vi "GDevCon Loops.vi"() -> ()   [LabVIEW 2020, in "CTI-Scratchpad.lvlib"]
uses:
  CTI-Scratchpad.lvlib
  CTI/Error Reporting.ctl
  CTI/GPIO Number.ctl
  CTI/I2C Number.ctl
  CTI/ADC Number.ctl
  CTI-Peripheral/Character LCD/Position.ctl
  CTI/GPIO Direction.ctl
  CTI/Raw ADC.ctl
  CTI-Peripheral/Grove I2C LCD/Grove I2C LCD.lvclass
  CTI/Session/Session.lvclass
  CTI/VisaComms/VisaComms.lvclass
  CTI/CTI.lvlib
  CTI-Peripheral/Character LCD/Char LCD.lvclass
panel:
  in  "Home":bool
  in  "Clear":bool
  in  "LED":bool
  in  "PWM Enable":bool
  out "Act. Freq":sgl format="%.4f"
  out "Act. Duty":sgl format="%_6f"
  in  "Frequency":sgl(slide) scale=10.0..500000.0
  in  "Duty":sgl(slide) scale=0.0..1.0
  out "Mic":dbl(knob) scale=0.0..4095.0
  out "PIR":bool
  out "Button":bool
  in  "Position":T1
  in  "Goto":bool
  out "Potentiometer":dbl(knob) scale=0.0..1.0
  in  "Write LCD":bool
  in  "LCD Text":string
  in  "Stop":bool
  in  "I2C Baud":u32=400000 format="%.0p"
  in  "Mic AI":T2=1
  in  "Pot AI":T2
  in  "SDA GPIO":T3=6
  in  "SCL GPIO":T3=7
  in  "I2C #":T4=1
  in  "PIR GPIO":T3=28
  in  "Buzzer GPIO":T3=18
  in  "LED GPIO":T3=20
  in  "Button GPIO":T3=16
  in  "Error Checking":T5
  in  "VISA resource name":refnum<visa-resource-name>="COM5"
  # "Buzzer"
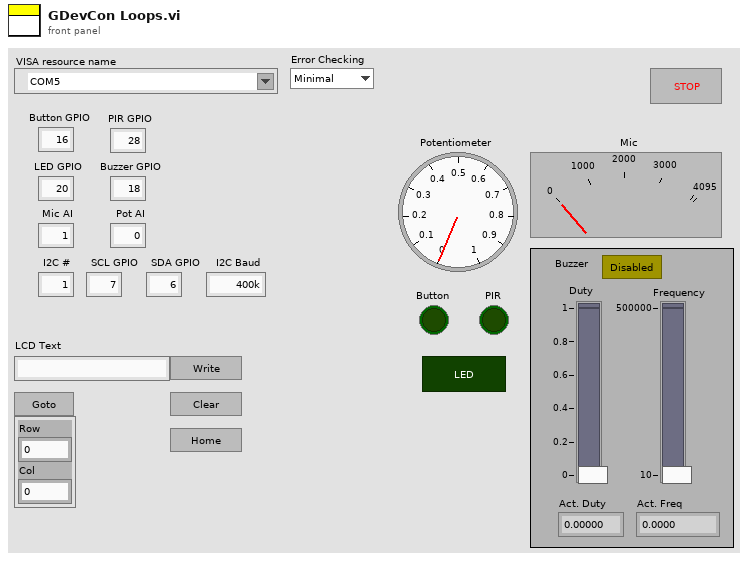
[diagram p1: front panel]
types:
  T1 = typedef "CTI-Peripheral.lvlib/Char LCD.lvclass/Position.ctl" = cluster{"Row":u8, "Col":u8}
  T2 = typedef "CTI.lvlib/ADC Number.ctl" = i8
  T3 = typedef "CTI.lvlib/GPIO Number.ctl" = i8
  T4 = typedef "CTI.lvlib/I2C Number.ctl" = i8
  T5 = typedef "CTI.lvlib/Error Reporting.ctl" = enum16{"Minimal", "Moderate", "Full"}
  T6 = typedef "CTI.lvlib/GPIO Direction.ctl" = enum16{"In", "Out"}
  T7 = typedef "CTI.lvlib/Raw ADC.ctl" = u16
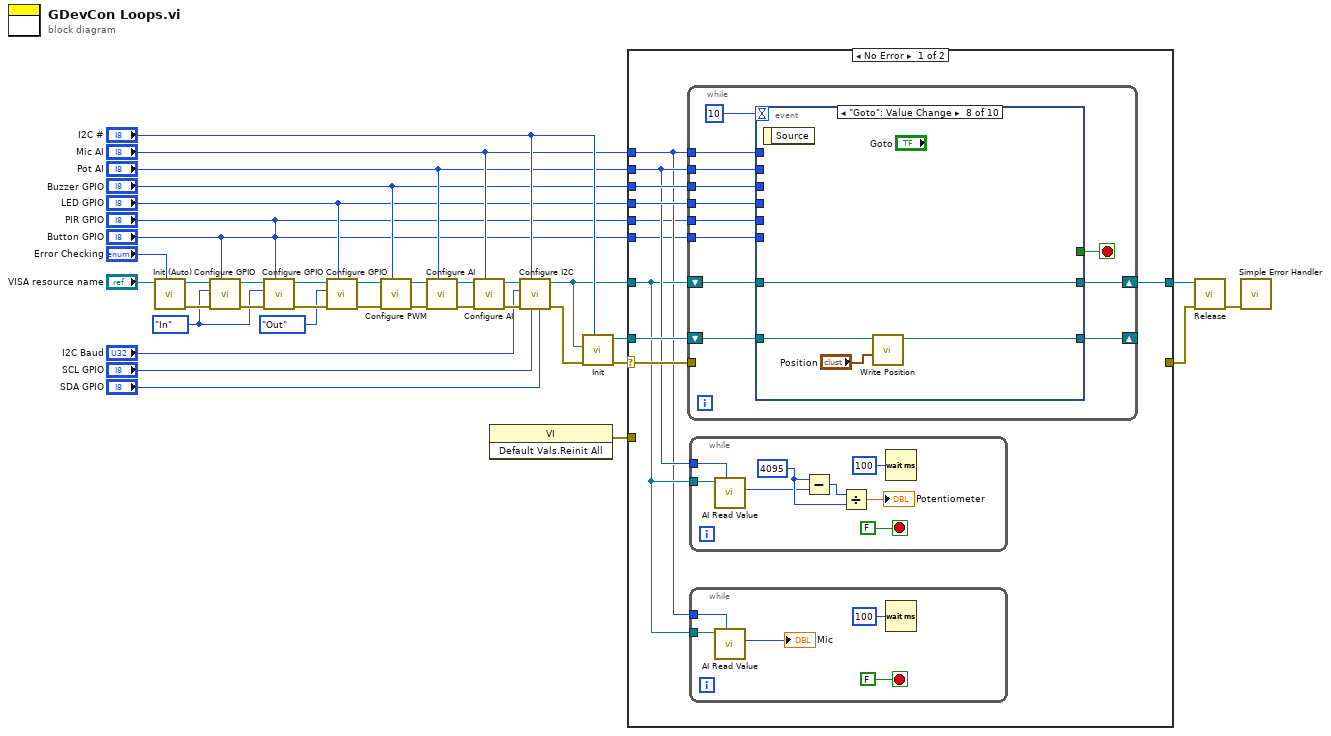
[diagram p0: block diagram]
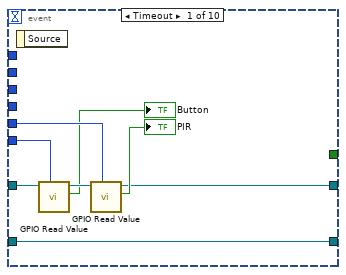
[diagram p2: hidden frame]
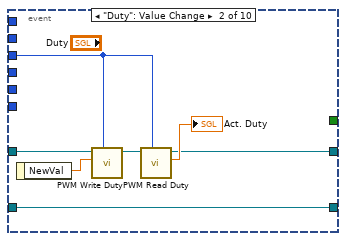
[diagram p3: hidden frame]
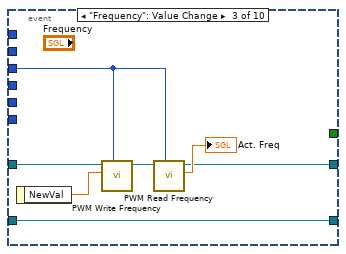
[diagram p4: hidden frame]
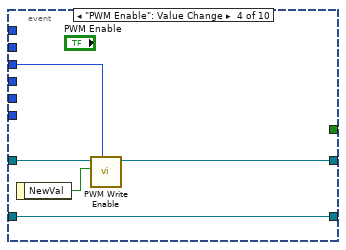
[diagram p5: hidden frame]
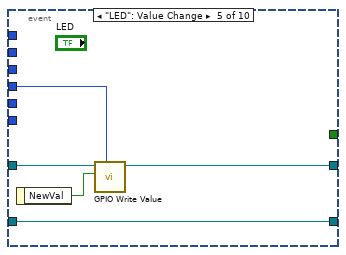
[diagram p6: hidden frame]
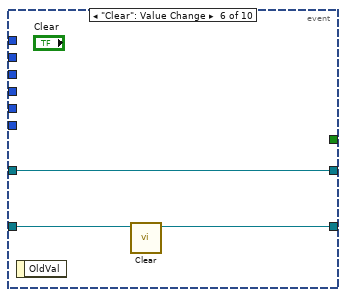
[diagram p7: hidden frame]
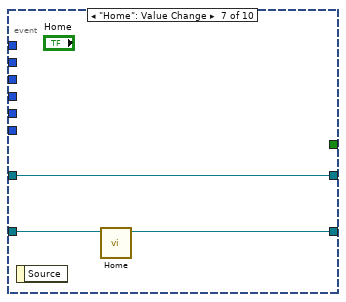
[diagram p8: hidden frame]
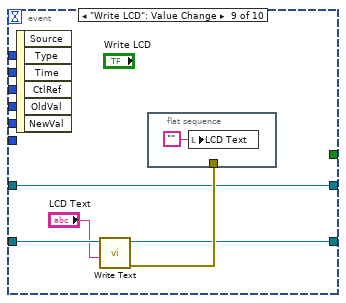
[diagram p9: hidden frame]
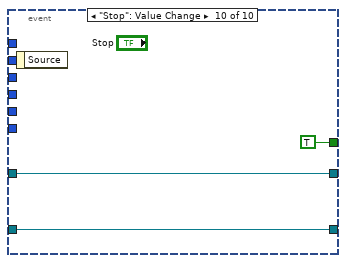
[diagram p10: hidden frame]
diagram:
  w26 = GPIO_Direction."In" ("GPIO Direction")
  n1 = call "Init (Auto).vi"("Error Checking (Full)"="Error Checking", "VISA resource name"="VISA resource name") -> ("error out"=w33:errorcluster, "Session"=w32:refnum<class "Session.lvclass">)  [unwired: 7 in, 1 out]
  n2 = call "Configure GPIO.vi"("GPIO #"="Button GPIO", "error in (no error)"=w33, "GPIO Direction"=w26, "Session in"=w32) -> ("error out"=w28:errorcluster, "Session out"=w27:refnum<class "Session.lvclass">)  [unwired: 6 in]
  n3 = call "Configure GPIO.vi"("GPIO #"="PIR GPIO", "error in (no error)"=w28, "GPIO Direction"=w26, "Session in"=w27) -> ("error out"=w36:errorcluster, "Session out"=w25:refnum<class "Session.lvclass">)  [unwired: 6 in]
  n4 = call "Configure GPIO.vi"("GPIO #"="LED GPIO", "error in (no error)"=w36, "GPIO Direction"=GPIO_Direction."Out", "Session in"=w25) -> ("error out"=w30:errorcluster, "Session out"=w31:refnum<class "Session.lvclass">)  [unwired: 6 in]
  n5 = call "Configure PWM.vi"("GPIO #"="Buzzer GPIO", "error in (no error)"=w30, "Session in"=w31) -> ("error out"=w20:errorcluster, "Session out"=w19:refnum<class "Session.lvclass">)  [unwired: 7 in]
  n6 = call "Configure AI.vi"("ADC #"="Pot AI", "error in (no error)"=w20, "Session in"=w19) -> ("error out"=w18:errorcluster, "Session out"=w17:refnum<class "Session.lvclass">)  [unwired: 7 in]
  n7 = call "Configure AI.vi"("ADC #"="Mic AI", "error in (no error)"=w18, "Session in"=w17) -> ("error out"=w15:errorcluster, "Session out"=w16:refnum<class "Session.lvclass">)  [unwired: 7 in]
  n8 = invoke class="VI" method="Default Vals.Reinit All"() -> (error out=w2:errorcluster)  [unwired: 3 in, 2 out]
  n9 = call "Configure I2C.vi"("SDA GPIO"="SDA GPIO", "SCL GPIO"="SCL GPIO", "I2C #"="I2C #", "error in (no error)"=w15, "Baud"="I2C Baud", "Session in"=w16) -> ("error out"=w23:errorcluster, "Session out"=w11:refnum<class "Session.lvclass">)  [unwired: 4 in]
  n10 = call "Init.vi"("I2C #"="I2C #", "error in (no error)"=w23, "Session In"=w11) -> ("error out"=w12:errorcluster, "Grove I2C LCD out"=w13:refnum<class "Grove I2C LCD.lvclass">)  [unwired: 7 in]
  n11 = case shown="No Error" w12 {
    selector: w12 -> [w45 w123]
    tunnel: w13 -> [w46 _]
    tunnel: w11 -> [w40 w124]
    tunnel: [w44 w124] -> w10
    tunnel: [_ w123] -> w9
    tunnel: "Mic AI" -> [w39 _]
    tunnel: "Pot AI" -> [w41 _]
    tunnel: "Buzzer GPIO" -> [w43 _]
    tunnel: "LED GPIO" -> [w42 _]
    tunnel: "PIR GPIO" -> [w37 _]
    tunnel: "Button GPIO" -> [_ _]
    tunnel: w2 -> [_ _]
    tunnel: "PIR GPIO" -> [w38 _]
    frame No Error {
      n12 = while {
        tunnel: w45 -> [_]
        shift-right: [w56] -> w44
        shift-left: w40 -> [w57]
        shift-right: [w55] -> _
        shift-left: w46 -> [w54]
        tunnel: w39 -> [w52]
        tunnel: w41 -> [w51]
        tunnel: w43 -> [w50]
        tunnel: w42 -> [w49]
        tunnel: w38 -> [w48]
        tunnel: w37 -> [w47]
        stop <- w53 stop-if-true
        n13 = event shown="[7] \"Goto\": Value Change" {
          selector: _ -> [_ _ _ _ _ _ _ _ _ _]
          dyn-events: _ -> [_ _ _ _ _ _ _ _ _ _]
          timeout: 10 -> [_ _ _ _ _ _ _ _ _ _]
          tunnel: w57 -> [w65 w72 w79 w84 w89 w93 w96 w100 w104 w109]
          tunnel: [w59 w68 w76 w81 w86 w93 w96 w100 w104 w109] -> w56
          tunnel: [w66 w73 w80 w85 w90 w92 w94 w97 w103 w108] -> w55
          tunnel: w54 -> [w66 w73 w80 w85 w90 w91 w95 w98 w102 w108]
          tunnel: [_ _ _ _ _ _ _ _ _ TRUE] -> w53
          tunnel: w52 -> [_ _ _ _ _ _ _ _ _ _]
          tunnel: w51 -> [_ _ _ _ _ _ _ _ _ _]
          tunnel: w50 -> [_ w67 w75 w82 _ _ _ _ _ _]
          tunnel: w49 -> [_ _ _ _ w87 _ _ _ _ _]
          tunnel: w48 -> [w62 _ _ _ _ _ _ _ _ _]
          tunnel: w47 -> [w64 _ _ _ _ _ _ _ _ _]
          event Timeout {
            n14 = event-data() -> ()  [unwired: 1 in, 1 out]
            n15 = call "GPIO Read Value.vi"("GPIO #"=w64, "Session in"=w65) -> ("Value"=→"Button":bool, "Session out"=w63:refnum<class "Session.lvclass">)  [unwired: 7 in, 1 out]
            n16 = call "GPIO Read Value.vi"("GPIO #"=w62, "Session in"=w63) -> ("Value"=→"PIR":bool, "Session out"=w59:refnum<class "Session.lvclass">)  [unwired: 7 in, 1 out]
          }
          event "Duty": Value Change {
            n17 = event-data() -> ("NewVal"=w71:sgl)  [unwired: 1 in]
            n18 = call "PWM Write Duty.vi"("GPIO #"=w67, "Duty % (0-1)"=w71, "Session in"=w72) -> ("Session out"=w70:refnum<class "Session.lvclass">)  [unwired: 7 in, 1 out]
            n19 = call "PWM Read Duty.vi"("GPIO #"=w67, "Session in"=w70) -> ("Duty % (0-1)"=→"Act. Duty":sgl, "Session out"=w68:refnum<class "Session.lvclass">)  [unwired: 7 in, 1 out]
          }
          event "Frequency": Value Change {
            n20 = event-data() -> ("NewVal"=w74:sgl)  [unwired: 1 in]
            n21 = call "PWM Write Frequency.vi"("GPIO #"=w75, "Frequency Hz"=w74, "Session in"=w79) -> ("Session out"=w78:refnum<class "Session.lvclass">)  [unwired: 7 in, 1 out]
            n22 = call "PWM Read Frequency.vi"("GPIO #"=w75, "Session in"=w78) -> ("Frequency Hz"=→"Act. Freq":sgl, "Session out"=w76:refnum<class "Session.lvclass">)  [unwired: 7 in, 1 out]
          }
          event "PWM Enable": Value Change {
            n23 = event-data() -> ("NewVal"=w83:bool)  [unwired: 1 in]
            n24 = call "PWM Write Enable.vi"("GPIO #"=w82, "Enable"=w83, "Session in"=w84) -> ("Session out"=w81:refnum<class "Session.lvclass">)  [unwired: 7 in, 1 out]
          }
          event "LED": Value Change {
            n25 = event-data() -> ("NewVal"=w88:bool)  [unwired: 1 in]
            n26 = call "GPIO Write Value.vi"("GPIO #"=w87, "Value"=w88, "Session in"=w89) -> ("Session out"=w86:refnum<class "Session.lvclass">)  [unwired: 7 in, 1 out]
          }
          event "Clear": Value Change {
            n27 = event-data() -> ()  [unwired: 1 in, 1 out]
            n28 = call-dynamic "Clear.vi"("Character LCD in"=w91) -> ("Character LCD out"=w92:refnum<class "Grove I2C LCD.lvclass">)  [unwired: 9 in, 1 out]
          }
          event "Home": Value Change {
            n29 = event-data() -> ()  [unwired: 1 in, 1 out]
            n30 = call-dynamic "Home.vi"("Character LCD in"=w95) -> ("Character LCD out"=w94:refnum<class "Grove I2C LCD.lvclass">)  [unwired: 9 in, 1 out]
          }
          event "Goto": Value Change {
            n31 = event-data() -> ()  [unwired: 1 in, 1 out]
            n32 = call-dynamic "Write Position.vi"("Position"="Position", "Grove I2C LCD I in"=w98) -> ("Grove I2C LCD I out"=w97:refnum<class "Grove I2C LCD.lvclass">)  [unwired: 8 in, 1 out]
          }
          event "Write LCD": Value Change {
            n33 = event-data() -> ()  [unwired: 1 in, 6 out]
            n34 = call-dynamic "Write Text.vi"("Text"="LCD Text", "Character LCD in"=w102) -> ("error out"=w105:errorcluster, "Character LCD out"=w103:refnum<class "Grove I2C LCD.lvclass">)  [unwired: 8 in]
            n35 = flat-sequence {
              tunnel: w105 -> [_]
              frame #0 {
                n36 = local write "LCD Text"("" ("LCD Text")) -> ()
              }
            }
          }
          event "Stop": Value Change {
            n37 = event-data() -> ()  [unwired: 1 in, 1 out]
          }
        }
      }
      n38 = while {
        tunnel: w40 -> [w122]
        tunnel: w41 -> [w121]
        stop <- FALSE stop-if-true
        w118 = T7 4095 ("y")
        n39 = call "AI Read Value.vi"("ADC #"=w121, "Session in"=w122) -> ("Value"=w117:T7)  [unwired: 7 in, 2 out]
        n40 = Subtract(x=w118, y=w117) -> (x-y=w120:T7)
        n41 = Divide(x=w120, y=w118) -> (x/y=→"Potentiometer":dbl)
        n42 = Wait (ms)(milliseconds to wait=u32 100) -> ()  [unwired: 1 out]
      }
      n43 = while {
        tunnel: w40 -> [w114]
        tunnel: w39 -> [w113]
        stop <- FALSE stop-if-true
        n44 = call "AI Read Value.vi"("ADC #"=w113, "Session in"=w114) -> ("Value"=→"Mic":T7)  [unwired: 7 in, 2 out]
        n45 = Wait (ms)(milliseconds to wait=u32 100) -> ()  [unwired: 1 out]
      }
    }
    frame Error {
    }
  }
  n46 = call-dynamic "Release.vi"("error in (no error)"=w9, "Session in"=w10) -> ("error out"=w8:errorcluster)  [unwired: 9 in]
  n47 = call <vilib>:"Simple Error Handler.vi"("error in (no error)"=w8) -> ()  [unwired: 4 in, 5 out]
